vi "IPS Initialize_Remote Unlocked.vi"(8 "Error In":errorcluster, 10 "Numeric":u32, 11 "VISA resource name (COM Port of Prologix Device)":refnum<visa-resource-name>="GPIB0::24::INSTR") -> ()   [LabVIEW 2013]
panel:
  out "Error Out":errorcluster={"status"=FALSE, "code"=1073676293, "source"="VISA Read in NI USB GPIB Command.vi->IPS Initialize_Remote Unlocked.vi"}
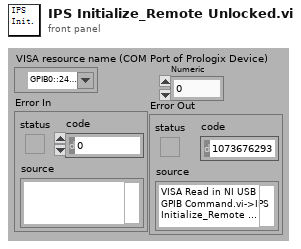
[diagram p1: front panel]
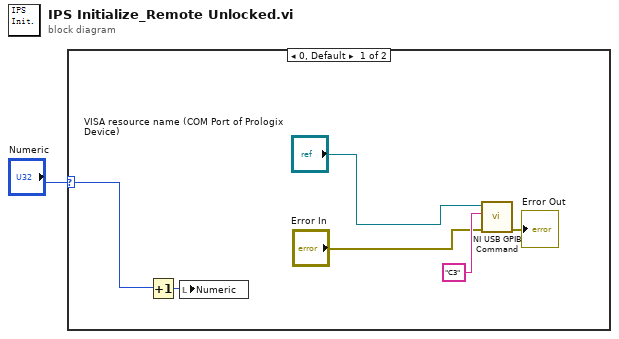
[diagram p0: block diagram]
diagram:
  n1 = case shown="0, Default" "Numeric" {
    selector: "Numeric" -> [w7 _]
    frame 0, Default {
      n2 = Increment(x=w7) -> (x+1=w6:u32)
      n3 = local write "Numeric"(w6) -> ()
      n4 = call "NI USB GPIB Command.vi"("Error In"="Error In", "String to Send"="C3", "VISA resource name"="VISA resource name (COM Port of Prologix Device)") -> ("Error Out"=→"Error Out":errorcluster)  [unwired: 1 in, 3 out]
    }
    frame 1 {
    }
  }
